vi "SVT Convert to RPM (analog).vi"(0 "tach signal [V]":waveform(dbl), 5 "tach info":T1={"threshold [V]"=1.0, "pulse width (2)"=2, "avg on n pulses (2)"=2, "pulse/revolution (1)"=1} {"pulse/revolution (1)" min=1 step=1; "avg on n pulses (2)" min=2 step=1; "pulse width (2)" min=1; "threshold [V]" format="%.2f"}, 11 "error in (no error)":errorcluster) -> (4 "rpm vs. time":cluster{"time [s]":dbl[], "speed [rpm]":dbl[]} {"speed [rpm]" format="%.2f"; "time [s]" format="%.2f"}, 6 "rpm vs. indices":cluster{"indices":dbl[], "speed [rpm]":dbl[]} {"speed [rpm]" format="%.2f"; "indices" format="%.2f"}, 15 "error out":errorcluster={"status"=TRUE, "code"=0, "source"=""})   [LabVIEW 2017]
doc: "Converts the signal acquired by a tachometer as a pulse train into a rotational speed expressed in revolutions per minute (rpm) versus time curve."
uses:
  <vilib>/Analysis/NI_AALPro.lvlib
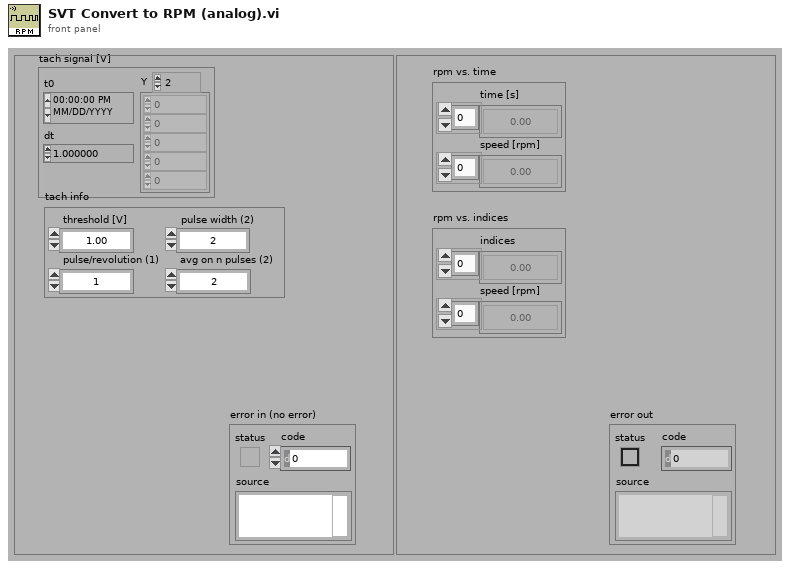
[diagram p1: front panel]
types:
  T1 = cluster{"threshold [V]":dbl, "pulse width (2)":i32, "avg on n pulses (2)":i32, "pulse/revolution (1)":i32}
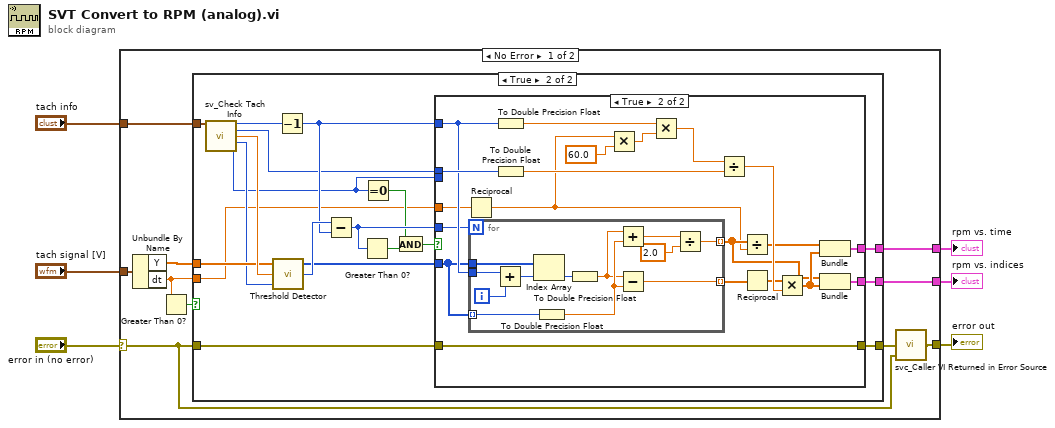
[diagram p0: block diagram]
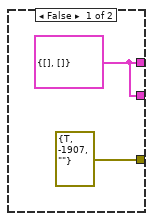
[diagram p2: hidden frame]
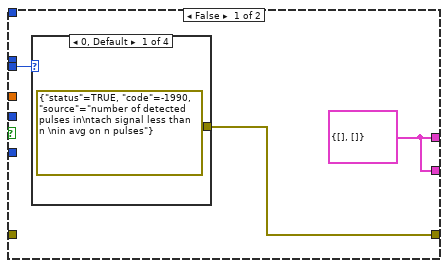
[diagram p3: hidden frame]
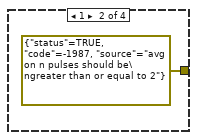
[diagram p4: hidden frame]
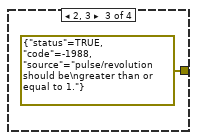
[diagram p5: hidden frame]
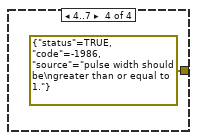
[diagram p6: hidden frame]
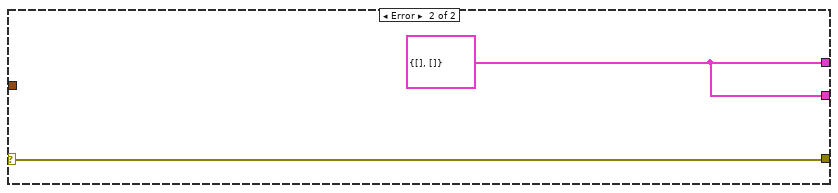
[diagram p7: hidden frame]
diagram:
  n1 = case shown="No Error" "error in (no error)" {
    selector: "error in (no error)" -> [w7 w78]
    tunnel: [w16 w77] -> w6
    tunnel: [w15 w77] -> w5
    tunnel: "tach info" -> [w14 _]
    tunnel: "tach signal [V]" -> [w13 _]
    tunnel: [w11 w78] -> w2
    frame No Error {
      n2 = Unbundle By Name(w13) -> ("Y"=w12:dbl[], "dt"=w9:dbl)
      n3 = Greater Than 0?(x=w9) -> (x > 0?=w8:bool)
      n4 = case shown="True" w8 {
        tunnel: [w17 w35] -> w16
        tunnel: [w17 w33] -> w15
        tunnel: w14 -> [_ w32]
        tunnel: w12 -> [_ w30]
        tunnel: w7 -> [_ w29]
        tunnel: [errorcluster {"status"=TRUE, "code"=-1907, "source"=""} ("error IO") w28] -> w10
        tunnel: w9 -> [_ w19]
        frame False {
          w17 = cluster{dbl[], dbl[]} {[], []}
        }
        frame True {
          n5 = call <vilib>:"sv_Check Tach Info.vi"("tach info"=w32) -> ("avg on n pulses"=w25:i32, "pulse/revolution (1)"=w24:i32, "threshold"=w31:dbl, "pulse width"=w26:i32, "error code"=w20:u32)  [unwired: 10 in]
          n6 = call <vilib>:"Threshold Detector.vi"("width"=w26, "threshold"=w31, "X"=w30) -> ("count"=w37:i32, "Indices"=w36:i32[])  [unwired: 1 out]
          n7 = Decrement(x=w25) -> (x-1=w27:i32)
          n8 = Subtract(x=w37, y=w27) -> (x-y=w34:i32)
          n9 = Greater Than 0?(x=w34) -> (x > 0?=w23:bool)
          n10 = Equal To 0?(x=w20) -> (x = 0?=w21:bool)
          n11 = And(x=w21, y=w23) -> (x .and. y?=w22:bool)
          n12 = case shown="True" w22 {
            tunnel: w34 -> [_ w51]
            tunnel: w24 -> [_ w63]
            tunnel: w27 -> [_ w59]
            tunnel: w36 -> [_ w57]
            tunnel: w19 -> [_ w46]
            tunnel: [w40 w52] -> w35
            tunnel: [w40 w50] -> w33
            tunnel: w29 -> [_ w48]
            tunnel: [w38 w48] -> w28
            tunnel: w20 -> [w39 _]
            frame False {
              w40 = cluster{dbl[], dbl[]} {[], []}
              n13 = case shown="0, Default" w39 {
                tunnel: [errorcluster {"status"=TRUE, "code"=-1990, "source"="number of detected pulses in\ntach signal less than n \nin avg on n pulses"} ("error IO") errorcluster {"status"=TRUE, "code"=-1987, "source"="avg on n pulses should be\ngreater than or equal to 2"} ("error IO") errorcluster {"status"=TRUE, "code"=-1988, "source"="pulse/revolution should be\ngreater than or equal to 1."} ("error IO") errorcluster {"status"=TRUE, "code"=-1986, "source"="pulse width should be\ngreater than or equal to 1."} ("error IO")] -> w38
                frame 0, Default {
                }
                frame 1 {
                }
                frame 2, 3 {
                }
                frame 4..7 {
                }
              }
            }
            frame True {
              n14 = Reciprocal(x=w46) -> (1/x=w45:dbl)
              n15 = for {
                N: w51 -> [_]
                tunnel: w57 -> [w76]
                tunnel: [w75] -> w62 mode=indexing
                tunnel: w57 -> [w72] mode=indexing
                tunnel: w59 -> [w73]
                tunnel: [w66] -> w47 mode=indexing
                i -> [w65]
                n16 = Add(x=w73, y=w65) -> (x+y=w74:i32)
                n17 = Index Array(array=w76, index=w74) -> (element=w71:i32)
                n18 = To Double Precision Float(number=w72) -> (double precision float=w69:dbl)
                n19 = To Double Precision Float(number=w71) -> (double precision float=w68:dbl)
                n20 = Add(x=w68, y=w69) -> (x+y=w70:dbl)
                n21 = Subtract(x=w68, y=w69) -> (x-y=w75:dbl)
                n22 = Divide(x=w70, y=2.0) -> (x/y=w66:dbl)
              }
              n23 = To Double Precision Float(number=w59) -> (double precision float=w54:dbl)
              n24 = To Double Precision Float(number=w63) -> (double precision float=w53:dbl)
              n25 = Multiply(x=w45, y=60.0) -> (x*y=w60:dbl)
              n26 = Multiply(x=w54, y=w60) -> (x*y=w58:dbl)
              n27 = Divide(x=w58, y=w53) -> (x/y=w64:dbl)
              n28 = Divide(x=w47, y=w45) -> (x/y=w56:dbl[])
              n29 = Reciprocal(x=w62) -> (1/x=w55:dbl[])
              n30 = Multiply(x=w55, y=w64) -> (x*y=w49:dbl[])
              n31 = Bundle(w56, w49) -> (w52:cluster{dbl[], dbl[]})  [unwired: 1 in]
              n32 = Bundle(w47, w49) -> (w50:cluster{dbl[], dbl[]})  [unwired: 1 in]
            }
          }
        }
      }
      n33 = call <vilib>:"svc_Caller VI Returned in Error Source.vi"("warning input to caller"=w7, "error in (no error)"=w10) -> ("error out"=w11:errorcluster)  [unwired: 3 in]
    }
    frame Error {
      w77 = cluster{dbl[], dbl[]} {[], []}
    }
  }
  "rpm vs. time" <- w6
  "rpm vs. indices" <- w5
  "error out" <- w2
